vi "Global 1.vi"() -> ()   [LabVIEW 2016]
panel:
  out "Numeric":dbl
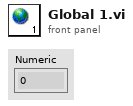
[diagram p1: front panel]
diagram:
